vi "Illini Hyperloop GUI v4.0.vi"() -> ()   [LabVIEW 2015]
uses:
  CommunicationStatus.ctl
  <vilib>/robotics/Controls/Attitude Indicator/Attitude Indicator.xctl
  StageEnum.ctl
  ArxPaxGauge4.ctl
  MicrosecondsGauge1.ctl
panel:
  out "RPM Right Front":T1 scale=0.0..6000.0
  out "RPM Right Mid":T1 scale=0.0..6000.0
  out "LEV Micro":T2 scale=800.0..2000.0
  out "RPM Right Back":T1 scale=0.0..6000.0
  out "RPM Left Front":T1 scale=0.0..6000.0
  out "RPM Left Mid":T1 scale=0.0..6000.0
  out "LEV  Delay timer":dbl
  out "STA  Delay timer":dbl
  out "Battery Pack 2 V 2":dbl(slide) caption="Capacity %" scale=0.0..100.0
  out "Battery Pack 1 V 2":dbl(slide) caption="Capacity %" scale=0.0..100.0
  out "Battery Pack 2 V":dbl(slide) caption="Pack 2 (V)" scale=0.0..500.0
  out "Battery Pack 1 V":dbl(slide) caption="Pack 1 (V)" scale=0.0..500.0
  out "Levitation Chart":cluster{"element":dbl, "element":dbl}(graph)
  out "Braking Force Chart 1":dbl(slide) caption="Reservoir 1" scale=0.0..6000.0
  out "Levitation height front":dbl(slide) caption="Front" scale=0.0..20.0
  out "Levitation height back":dbl(slide) caption="Back" scale=0.0..20.0
  out "Current front right":dbl[unit] caption="Current"
  out "Voltage front right":dbl[unit] caption="Voltage"
  out "Current front left":dbl[unit] caption="Current"
  out "Voltage front left":dbl[unit] caption="Voltage"
  out "Current back right":dbl[unit] caption="Current"
  out "Voltage back right":dbl[unit] caption="Voltage"
  out "Current back left":dbl[unit] caption="Current"
  out "Voltage back left":dbl[unit] caption="Voltage"
  out "Attitude Indicator":cluster{"Roll":dbl, "Pitch":dbl}(xcontrol)
  out "Yaw":dbl(knob) scale=-15.0..15.0
  out "RPM Left Back":T1 scale=0.0..6000.0
  out "Cabin Pressure":dbl format="%#.3g"
  out "Ambient Pressure (psi)":dbl(graph)
  out "Pod State:":T3
  out "Communication Status:":T4
  out "Low Battery":dbl format="%#.2g"
  out "High Battery:":dbl format="%#.2g"
  out "Battery 3":dbl(slide) scale=0.0..100.0
  out "Battery 2":dbl(slide) scale=0.0..100.0
  out "Battery 1":dbl(slide) scale=0.0..100.0
  out "Z acc":dbl
  out "Y acc":dbl
  out "X acc":dbl
  out "Z vel":dbl
  out "Y vel":dbl
  out "X vel":dbl
  out "Z position":dbl
  out "Y pos":dbl
  out "X pos":dbl
  out "Velocity Chart":dbl(graph)
  in  "EMERGENCY BRAKE":bool
  in  "Functional Test Tab Control":T5(tab)
  out "Client Closed":string="The client VI closed the connection."
  out "Most Recent Data":string
  in  "Connect to":string="192.168.137.100"
  in  "timeout ms":i32=1000
  in  "port":u16=8888
  in  "ms per loop":u32
  in  "bytes per write":i32=1000
  out "Base File Name":string
  in  "Transition":bool
  in  "Transition to:":string(combo)="Safe Mode"
  out "bytes written":i32
  in  "Stop Program":bool
  out "Producer Error Messages":errorcluster
  out "Consumer Error Messages":errorcluster
  in  "LEV OFF":bool
  in  "STA Delay":dbl=100.0
  in  "LEV Delay":dbl=100.0
  in  "STA Start Stop":bool
  in  "LEV Start Stop":bool
  in  "STA jump Interval":dbl=5.0
  in  "STA Target":dbl=1000.0
  in  "LEV jump interval":dbl=5.0
  in  "LEV Target":dbl=1000.0
  in  "STA Init + Arm":bool
  in  "STA init":dbl
  in  "STA arm":dbl
  in  "LEV ON":bool
  in  "SET STA Manual":bool
  in  "Set LEV Manual":bool
  in  "LEV SLIDE":dbl(slide) scale=0.0..2000.0
  in  "STA Slide":dbl(slide) scale=0.0..2000.0
  in  "STA Margin":dbl=50.0
  in  "LEV Margin":dbl=50.0
  out "Functional Test C Data":string caption="Data:"
  in  "Functional Test 3":bool caption="Boolean"
  in  "Functional Test 4":bool caption="Boolean"
  out "Functional Test D Data":string caption="Data:"
  in  "Prepare for Launch":bool caption="Boolean"
  out "Acceleration Chart":dbl(graph)
  out "Checkmark":u16(ring)
  out "Position Chart":dbl(graph)
  out "Temperature other (C)":T6(graph)
  out "Temperature ESCs (C)":T7(graph)
  # "Illini Hyperloop"
  # "Brakes (PSI)"
  # "X Position (m)"
  # "Levitation (m)"
  # "Attitude"
  # "Levitation (mm)"
  # "X Acceleration (m/s/s)"
  # "X Velocity (m/s)"
  # "Levitation Battery Packs"
  # "Motor Control"
  # "Brake Control"
  # "Functional Test C: Communication Inside Tube"
  # "Functional Test D: Internal power and Levitation"
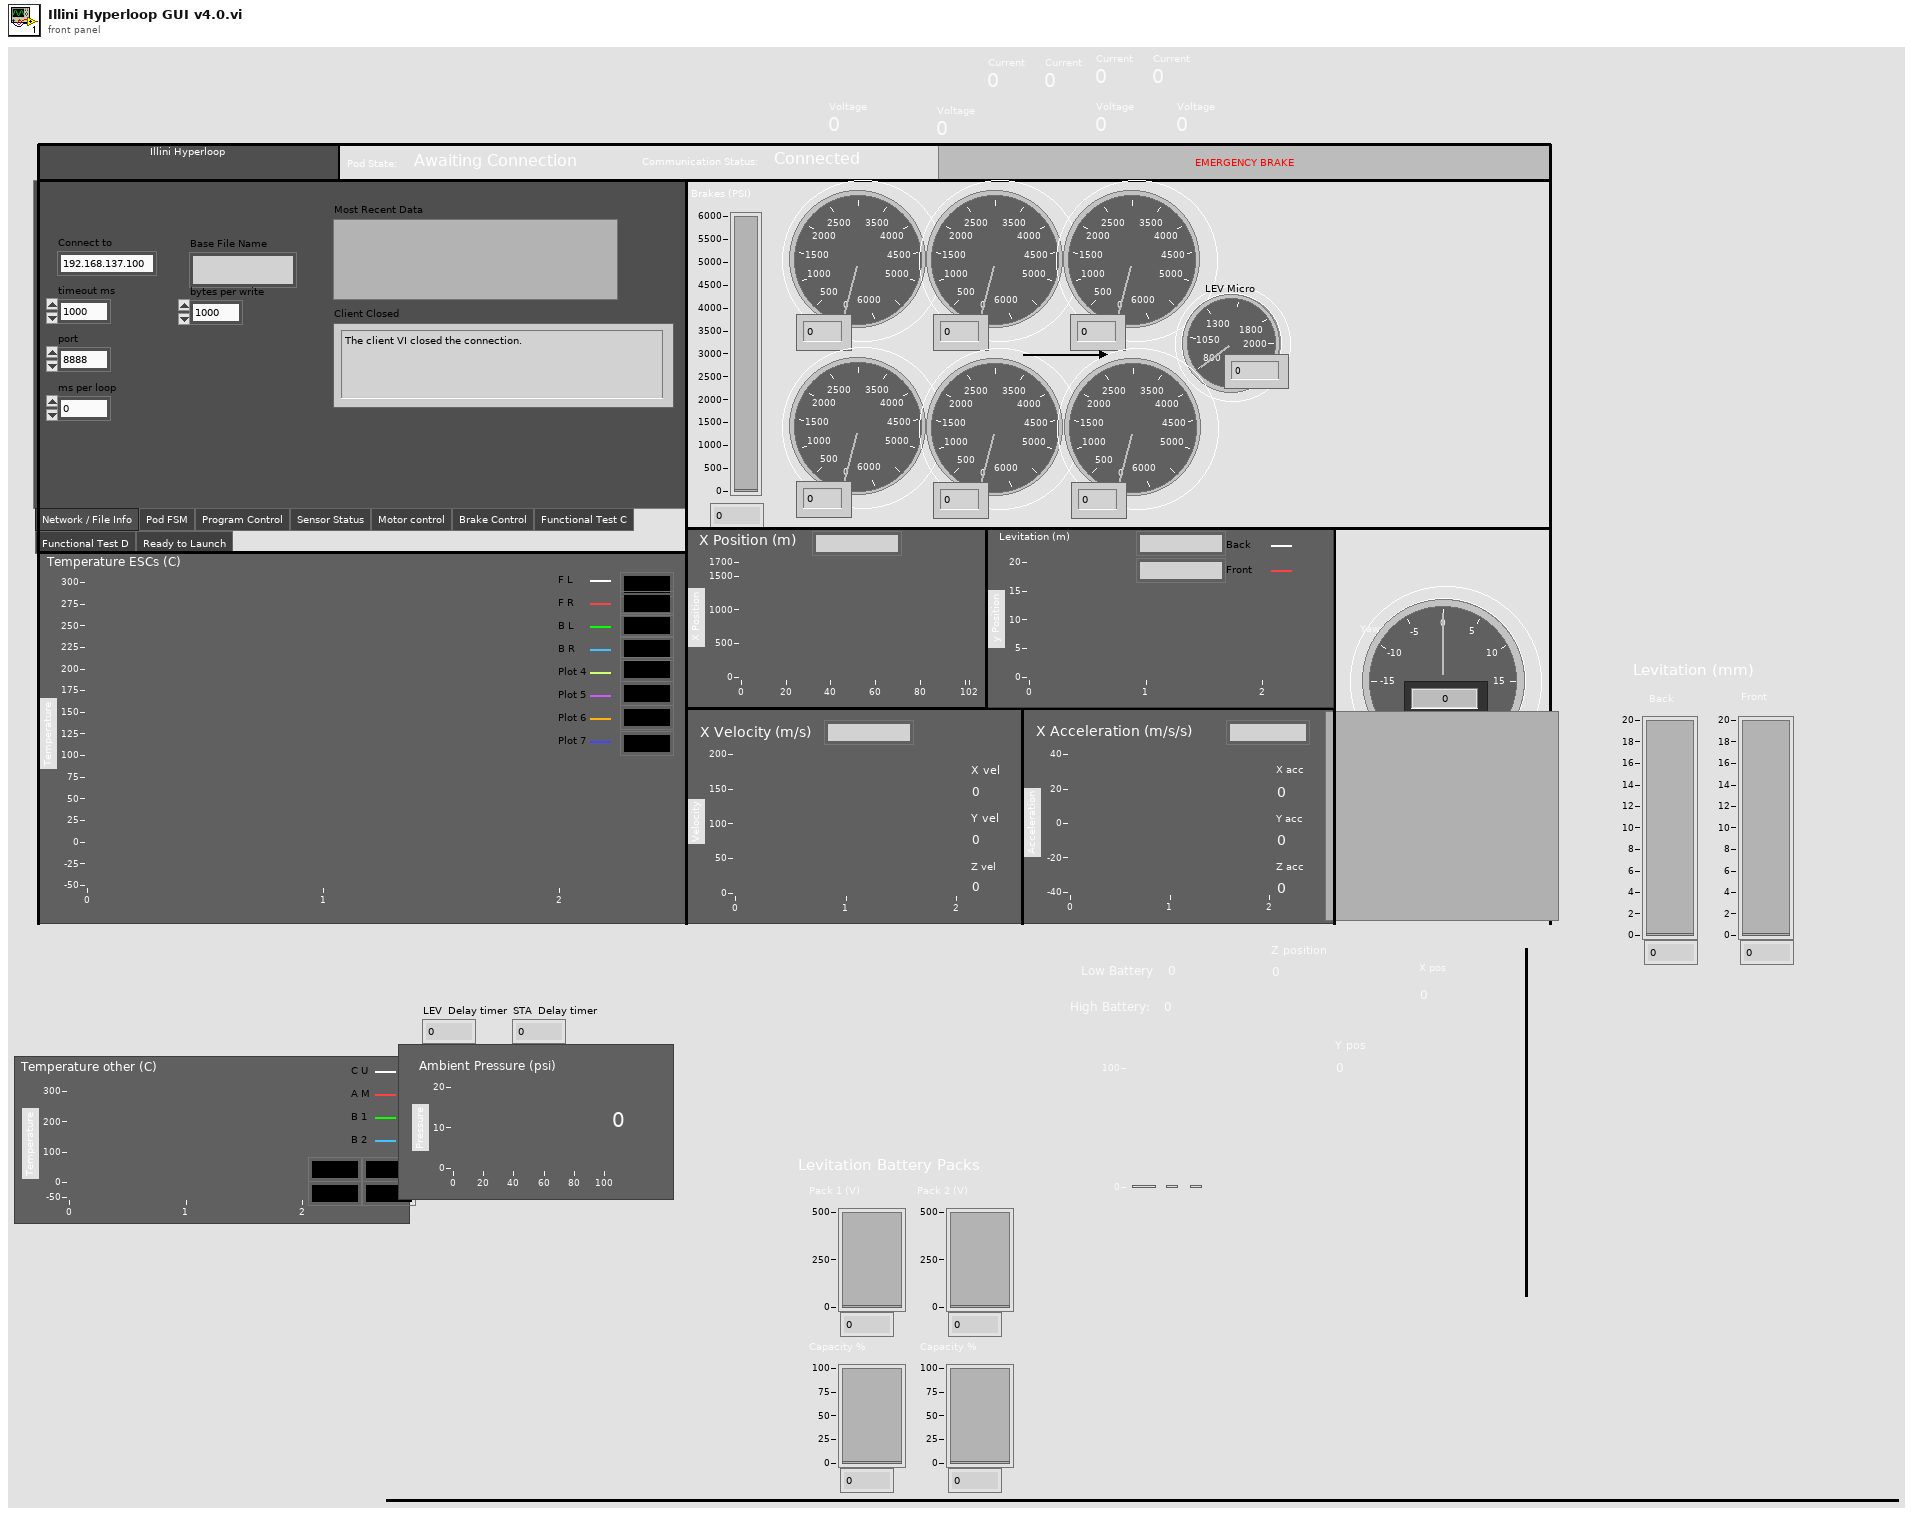
[diagram p1: front panel]
types:
  T1 = typedef "ArxPaxGauge4.ctl" = u32
  T2 = typedef "MicrosecondsGauge1.ctl" = dbl
  T3 = typedef "StageEnum.ctl" = enum16{"Awaiting Connection", "TEST Comms", "TEST Lev", "TEST Inside Comms", "TEST Internal Power", "Ready to Launch", "Acceleration", "Coast", "Brake"}
  T4 = typedef "CommunicationStatus.ctl" = enum16{"Connected", "Disconnected"}
  T5 = enum32{"Network / File Info", "Pod FSM", "Program Control", "Sensor Status", "Motor control", "Brake Control", "Functional Test C", "Functional Test D", "Ready to Launch"}
  T6 = cluster{"element":dbl, "element":dbl, "element":dbl, "element":dbl}
  T7 = cluster{"element":dbl, "element":dbl, "element":dbl, "element":dbl, "element":dbl, "element":dbl, "element":dbl, "element":dbl}
  T8 = cluster{"element":dbl, "element":dbl, "element":dbl, "element":dbl, "element":dbl, "element":dbl, "element":dbl, "element":dbl}[]
  T9 = cluster{"element":dbl, "element":dbl, "element":dbl, "element":dbl}[]
  T10 = enum16{"Standard", "Buffered", "CRLF", "Immediate"}
  T11 = cluster{i32, "data out":string, "data out":string}
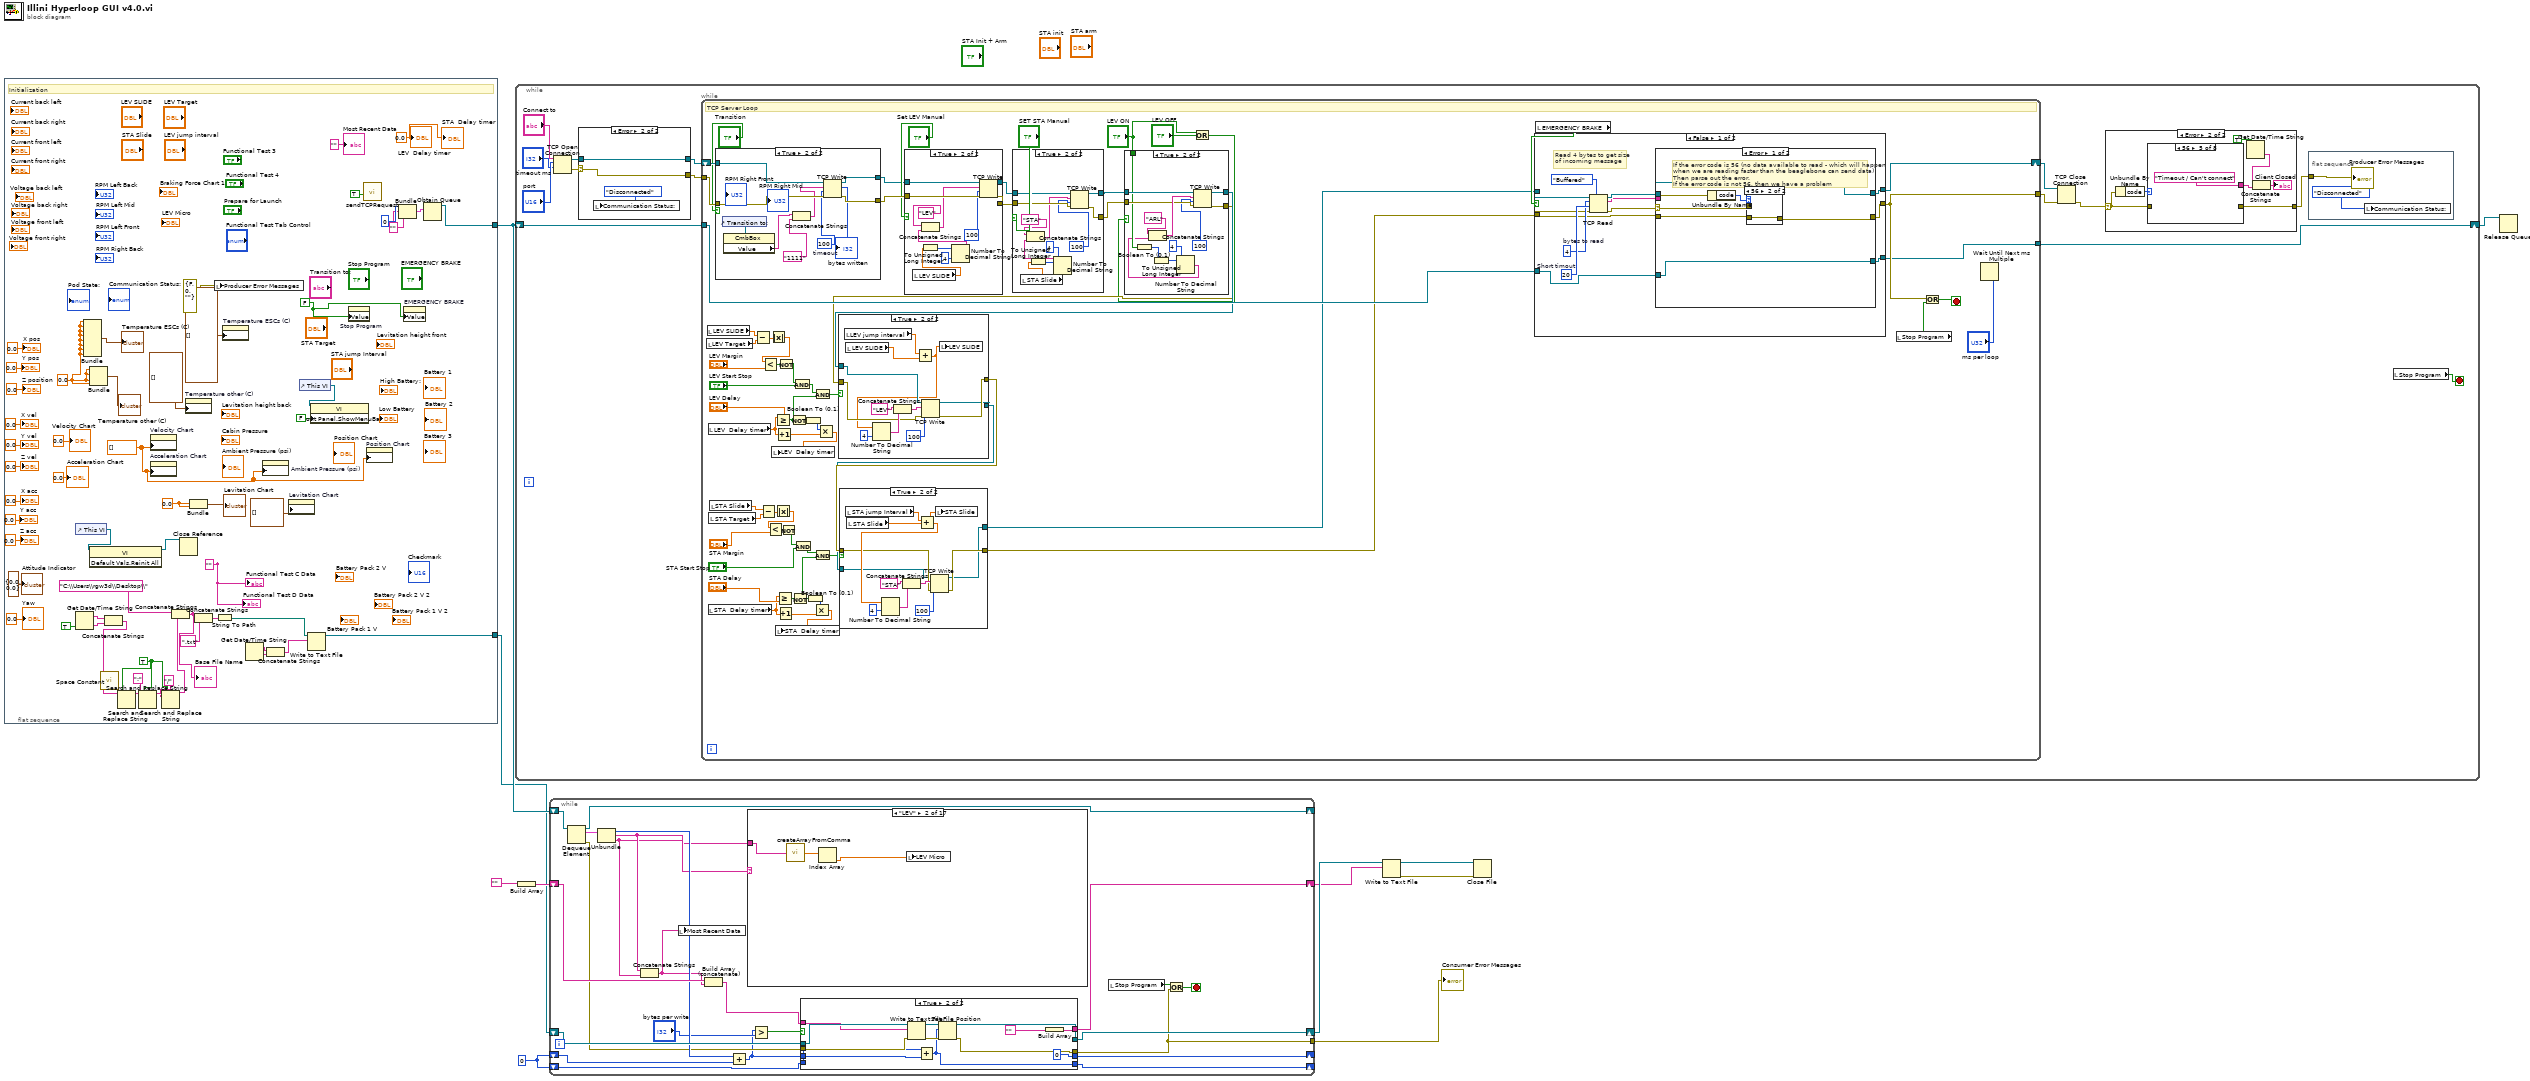
[diagram p0: block diagram]
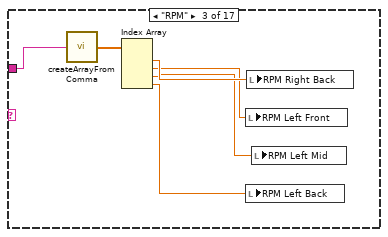
[diagram p4: hidden frame]
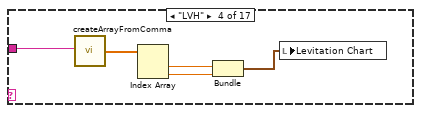
[diagram p5: hidden frame]
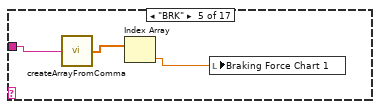
[diagram p6: hidden frame]
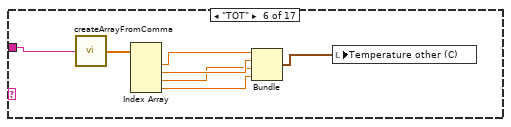
[diagram p7: hidden frame]
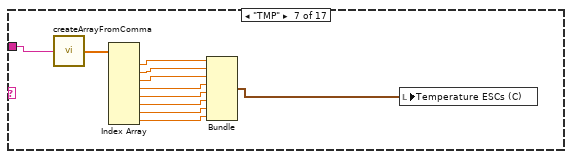
[diagram p8: hidden frame]
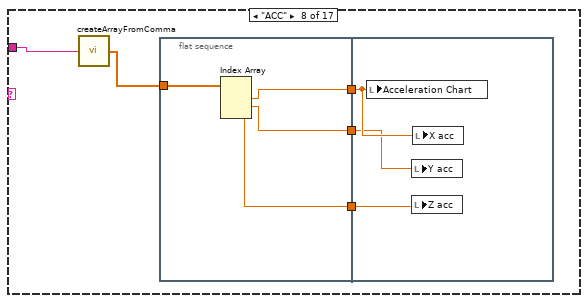
[diagram p9: hidden frame]
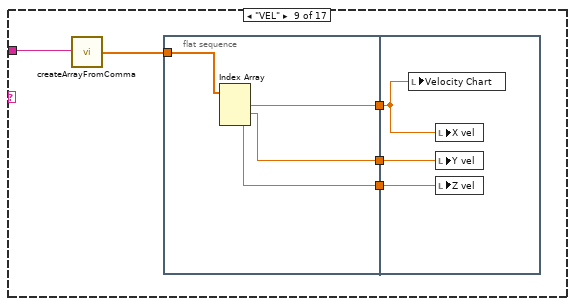
[diagram p10: hidden frame]
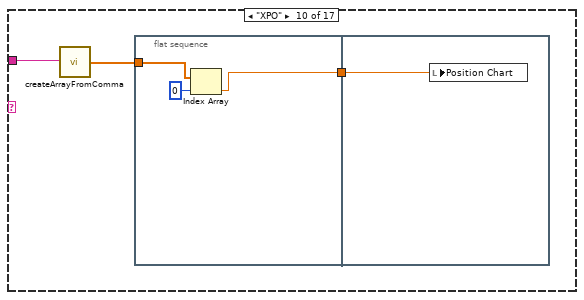
[diagram p11: hidden frame]
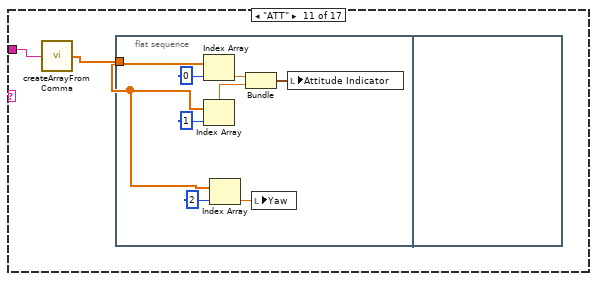
[diagram p12: hidden frame]
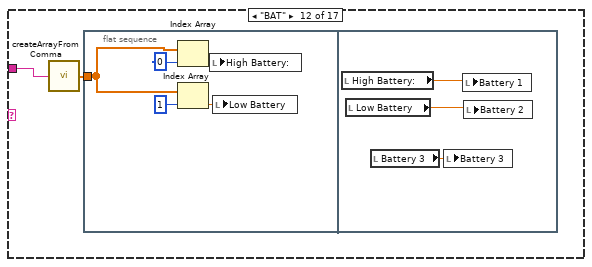
[diagram p13: hidden frame]
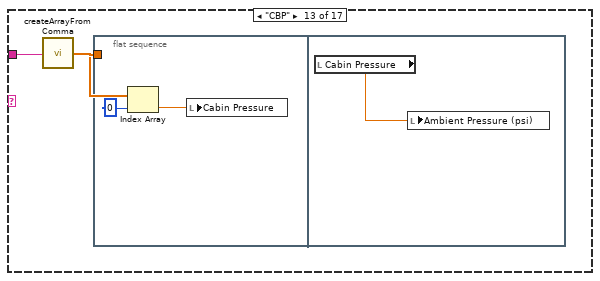
[diagram p14: hidden frame]
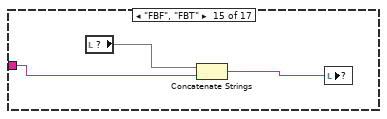
[diagram p16: hidden frame]
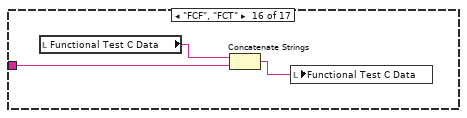
[diagram p17: hidden frame]
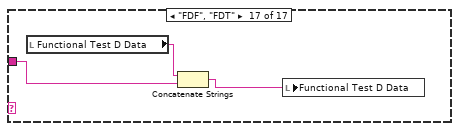
[diagram p18: hidden frame]
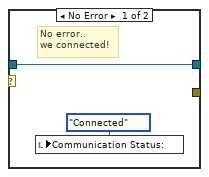
[diagram p19: hidden frame]
diagram:
  w1 = 0
  n1 = flat-sequence {
    tunnel: [w67] -> w11
    tunnel: [w40] -> w6
    frame #0 {
      w19 = 0.0 ("LEV  Delay timer")
      w23 = 0.0 ("element")
      w24 = TRUE ("want seconds? (F)")
      w37 = ""
      w44 = dbl[] [] ("History Data")
      w18 = 0.0 ("element")
      w52 = FALSE
      w20 = "" ("Functional Test 1 Data")
      # "Initialization"
      n2 = control-ref of="This VI"() -> (w46:refnum<vi>)
      n3 = Get Date/Time String(want seconds? (F)=TRUE) -> (date string=w35:string, time string=w34:string)  [unwired: 2 in]
      n4 = Bundle("element"=w18, "element"=w18, "element"=w18, "element"=w18, "element"=w18, "element"=w18, "element"=w18, "element"=w18) -> (→"Temperature ESCs (C)":T7)  [unwired: 1 in]
      n5 = Bundle("element"=w18, "element"=w18, "element"=w18, "element"=w18) -> (→"Temperature other (C)":T6)  [unwired: 1 in]
      n6 = invoke class="VI" method="Default Vals.Reinit All"(reference=w46) -> (reference out=w45:refnum<vi>)  [unwired: 2 in, 2 out]
      n7 = call <vilib>:"Space Constant.vi"() -> ("String"=w36:string)
      n8 = Concatenate Strings(w35, w34) -> (w33:string)
      n9 = Search and Replace String(replace all?=w24, input string=w33, search string=w36) -> (result string=w31:string)  [unwired: 5 in, 3 out]
      n10 = Search and Replace String(replace all?=w24, input string=w31, search string=":" ("Functional Test 1 Data")) -> (result string=w27:string)  [unwired: 5 in, 3 out]
      n11 = property on="Velocity Chart" class="WFChart (strict)"("History Data"=w44) -> ()  [unwired: 2 in, 2 out]
      n12 = property on="Acceleration Chart" class="WFChart (strict)"("History Data"=w44) -> ()  [unwired: 2 in, 2 out]
      n13 = Search and Replace String(replace all?=w24, input string=w27, search string="/" ("Functional Test 1 Data")) -> (result string=w26:string)  [unwired: 5 in, 3 out]
      n14 = Concatenate Strings("C:\\Users\\rgw3d\\Desktop\\" ("Functional Test 1 Data"), w26) -> (w13:string)
      "Base File Name" <- w13
      n15 = Close Reference(reference=w45) -> ()  [unwired: 1 in, 1 out]
      n16 = property on="Temperature other (C)" class="WFChart (strict)"("History Data"=T9 []) -> ()  [unwired: 2 in, 2 out]
      n17 = Bundle("element"=w23, "element"=w23) -> (→"Levitation Chart":cluster{"element":dbl, "element":dbl})  [unwired: 1 in]
      n18 = Concatenate Strings(w13, ".txt" ("Functional Test 1 Data")) -> (w14:string)
      n19 = local write "Producer Error Messages"(errorcluster {"status"=FALSE, "code"=0, "source"=""} ("error constant")) -> ()
      n20 = String To Path(string=w14) -> (path=w28:path)
      n21 = property on="Temperature ESCs (C)" class="WFChart (strict)"("History Data"=T8 []) -> ()  [unwired: 2 in, 2 out]
      n22 = Get Date/Time String() -> (date string=w43:string, time string=w42:string)  [unwired: 3 in]
      n23 = property on="Ambient Pressure (psi)" class="WFChart (strict)"("History Data"=w44) -> ()  [unwired: 2 in, 2 out]
      n24 = Concatenate Strings(w43, w42) -> (w41:string)
      n25 = property on="Levitation Chart" class="WFChart (strict)"("History Data"=cluster{"element":dbl, "element":dbl}[] []) -> ()  [unwired: 2 in, 2 out]
      n26 = control-ref of="This VI"() -> (w51:refnum<vi>)
      n27 = Write to Text File(file (use dialog)=w28, text=w41) -> (refnum out=w40:refnum<file>)  [unwired: 2 in, 2 out]
      n28 = property class="VI"(reference=w51, "Front Panel.ShowMenuBar"=FALSE ("Front Panel Window:Show Menu Bar")) -> ()  [unwired: 1 in, 2 out]
      n29 = property on="Stop Program" class="Bool (strict)"("Value"=w52) -> ()  [unwired: 2 in, 2 out]
      n30 = call "sendTCPRequest.vi"("Force Reset"=TRUE) -> ()  [unwired: 9 in, 2 out]
      n31 = property on="Position Chart" class="WFChart (strict)"("History Data"=w44) -> ()  [unwired: 2 in, 2 out]
      n32 = Bundle(0, w37, w37) -> (w39:cluster{i32, string, string})  [unwired: 1 in]
      n33 = property on="EMERGENCY BRAKE" class="Bool (strict)"("Value"=w52) -> ()  [unwired: 2 in, 2 out]
      n34 = Obtain Queue(element data type=w39) -> (queue out=w67:refnum<queue>)  [unwired: 4 in, 2 out]
      "X pos" <- 0.0 ("X position")
      "Y pos" <- 0.0 ("Y position")
      "Z position" <- 0.0 ("Z position")
      "X vel" <- 0.0 ("X velocity")
      "Y vel" <- 0.0 ("Y velocity")
      "Z vel" <- 0.0 ("Z velocity")
      "X acc" <- 0.0 ("X acceleration")
      "Y acc" <- 0.0 ("Y acceleration")
      "Z acc" <- 0.0 ("Z acceleration")
      "Velocity Chart" <- 0.0 ("Velocity (m/s)")
      "Attitude Indicator" <- cluster{"Roll":dbl, "Pitch":dbl} {"Roll"=0.0, "Pitch"=0.0} ("Attitude Indicator")
      "Acceleration Chart" <- 0.0 ("Acceleration Chart")
      "Yaw" <- 0.0 ("Yaw")
      "Functional Test C Data" <- w20
      "Functional Test D Data" <- w20
      "Most Recent Data" <- "" ("Data out")
      "LEV  Delay timer" <- w19
      "STA  Delay timer" <- w19
    }
  }
  n35 = while {
    shift-right: [w74] -> w10
    shift-left: w11 -> [w75]
    stop <- w71 stop-if-true
    n36 = TCP Open Connection(address="Connect to", remote port or service name="port", timeout ms (60000)="timeout ms") -> (connection ID=w76:refnum<k5>, error out=w77:errorcluster)  [unwired: 2 in]
    n37 = case shown="Error" w77 {
      selector: w77 -> [_ w87]
      tunnel: w76 -> [w85 w88]
      tunnel: [w85 w88] -> w69
      tunnel: [_ w87] -> w68
      frame No Error {
        # "No error.. \nwe connected!"
        n38 = local write "Communication Status:"(CommunicationStatus."Connected" ("Communication Status")) -> ()
      }
      frame Error {
        n39 = local write "Communication Status:"(CommunicationStatus."Disconnected" ("Communication Status")) -> ()
      }
    }
    n40 = while {
      tunnel: w68 -> [w160]
      tunnel: [w165] -> w73
      tunnel: w75 -> [w155]
      tunnel: [w164] -> w74
      shift-right: [w163] -> w70
      shift-left: w69 -> [w161]
      stop <- w154 stop-if-true
      # "TCP Server Loop"
      n41 = local read "LEV Target"() -> (w149:dbl)
      n42 = local read "LEV SLIDE"() -> (w150:dbl)
      n43 = local read "LEV  Delay timer"() -> (w133:dbl)
      n44 = local read "STA  Delay timer"() -> (w132:dbl)
      n45 = local read "STA Target"() -> (w143:dbl)
      n46 = local read "STA Slide"() -> (w144:dbl)
      n47 = case shown="True" "Transition" {
        tunnel: w161 -> [w237 w247]
        tunnel: w160 -> [w236 w245]
        tunnel: [w236 w244] -> w158
        tunnel: [w237 w246] -> w156
        frame False {
        }
        frame True {
          w243 = 100  # timeout
          n48 = control-ref of="Transition to:"() -> (w242:refnum<vi>)
          n49 = property class="CmbBox"(reference=w242) -> ("Value"=w240:string)  [unwired: 1 in, 2 out]
          n50 = Concatenate Strings(w240, "1111") -> (w238:string)
          n51 = TCP Write(connection ID=w247, data in=w238, error in (no error)=w245, 9:w243) -> (connection ID out=w246:refnum<k5>, bytes written=→"bytes written":i32, error out=w244:errorcluster)
        }
      }
      n52 = Subtract(x=w150, y=w149) -> (x-y=w148:dbl)
      n53 = Subtract(x=w144, y=w143) -> (x-y=w146:dbl)
      n54 = Absolute Value(x=w148) -> (abs(x)=w147:dbl)
      n55 = Less?(x=w147, y="LEV Margin") -> (x < y?=w124:bool)
      n56 = Greater Or Equal?(x=w133, y="LEV Delay") -> (x >= y?=w121:bool)
      n57 = Absolute Value(x=w146) -> (abs(x)=w145:dbl)
      n58 = Less?(x=w145, y="STA Margin") -> (x < y?=w115:bool)
      n59 = Increment(x=w133) -> (x+1=w130:dbl)
      n60 = Greater Or Equal?(x=w132, y="STA Delay") -> (x >= y?=w113:bool)
      n61 = Increment(x=w132) -> (x+1=w118:dbl)
      n62 = Not(x=w124) -> (.not. x?=w122:bool)
      n63 = Not(x=w115) -> (.not. x?=w116:bool)
      n64 = Not(x=w121) -> (.not. x?=w131:bool)
      n65 = Not(x=w113) -> (.not. x?=w126:bool)
      n66 = And(x=w122, y="LEV Start Stop") -> (x .and. y?=w120:bool)
      n67 = And(x=w116, y="STA Start Stop") -> (x .and. y?=w136:bool)
      n68 = Boolean To (0,1)(Boolean=w131) -> (0, 1=w128:i16)
      n69 = Boolean To (0,1)(Boolean=w126) -> (0, 1=w125:i16)
      n70 = Multiply(x=w125, y=w118) -> (x*y=w127:dbl)
      n71 = local write "STA  Delay timer"(w127) -> ()
      n72 = And(x=w120, y=w121) -> (x .and. y?=w134:bool)
      n73 = And(x=w136, y=w113) -> (x .and. y?=w135:bool)
      n74 = Multiply(x=w128, y=w130) -> (x*y=w129:dbl)
      n75 = local write "LEV  Delay timer"(w129) -> ()
      n76 = case shown="True" "Set LEV Manual" {
        tunnel: w158 -> [w223 w235]
        tunnel: [w223 w234] -> w152
        tunnel: w156 -> [w224 w233]
        tunnel: [w224 w232] -> w153
        frame False {
        }
        frame True {
          n77 = local read "LEV SLIDE"() -> (w226:dbl)
          n78 = To Unsigned Long Integer(number=w226) -> (unsigned 32bit integer=w225:u32)
          n79 = Number To Decimal String(number=w225, width (-)=i16 4) -> (decimal integer string=w229:string)
          n80 = Concatenate Strings("LEV", w229) -> (w228:string)
          n81 = TCP Write(connection ID=w233, data in=w228, error in (no error)=w235, 9:100 ("timeout ms (25000)")) -> (connection ID out=w232:refnum<k5>, error out=w234:errorcluster)  [unwired: 1 out]
        }
      }
      n82 = case shown="True" "SET STA Manual" {
        tunnel: w153 -> [w211 w222]
        tunnel: [w211 w221] -> w112
        tunnel: w152 -> [w210 w220]
        tunnel: [w210 w219] -> w111
        frame False {
        }
        frame True {
          n83 = local read "STA Slide"() -> (w212:dbl)
          n84 = To Unsigned Long Integer(number=w212) -> (unsigned 32bit integer=w213:u32)
          n85 = Number To Decimal String(number=w213, width (-)=i16 4) -> (decimal integer string=w216:string)
          n86 = Concatenate Strings("STA", w216) -> (w215:string)
          n87 = TCP Write(connection ID=w222, data in=w215, error in (no error)=w220, 9:100 ("timeout ms (25000)")) -> (connection ID out=w221:refnum<k5>, error out=w219:errorcluster)  [unwired: 1 out]
        }
      }
      n88 = Or(x="LEV ON", y="LEV OFF") -> (x .or. y?=w107:bool)
      n89 = case shown="True" w107 {
        tunnel: w112 -> [w168 w178]
        tunnel: w111 -> [w169 w177]
        tunnel: [w169 w176] -> w109
        tunnel: [w168 w175] -> w110
        tunnel: "LEV ON" -> [_ w172]
        frame False {
        }
        frame True {
          n90 = Boolean To (0,1)(Boolean=w172) -> (0, 1=w173:i16)
          n91 = To Unsigned Long Integer(number=w173) -> (unsigned 32bit integer=w179:u32)
          n92 = Number To Decimal String(number=w179, width (-)=i16 4) -> (decimal integer string=w170:string)
          n93 = Concatenate Strings("ARL", w170) -> (w181:string)
          n94 = TCP Write(connection ID=w178, data in=w181, error in (no error)=w177, 9:100 ("timeout ms (25000)")) -> (connection ID out=w175:refnum<k5>, error out=w176:errorcluster)  [unwired: 1 out]
        }
      }
      n95 = case shown="True" w134 {
        tunnel: w110 -> [w197 w203]
        tunnel: [w197 w199] -> w140
        tunnel: w109 -> [w196 w202]
        tunnel: [w196 w201] -> w142
        frame False {
        }
        frame True {
          n96 = local read "LEV jump interval"() -> (w209:dbl)
          n97 = local read "LEV SLIDE"() -> (w208:dbl)
          n98 = Add(x=w209, y=w208) -> (x+y=w200:dbl)
          n99 = Number To Decimal String(number=w200, width (-)=i16 4) -> (decimal integer string=w205:string)
          n100 = Concatenate Strings("LEV", w205) -> (w207:string)
          n101 = TCP Write(connection ID=w203, data in=w207, error in (no error)=w202, 9:100 ("timeout ms (25000)")) -> (connection ID out=w199:refnum<k5>, error out=w201:errorcluster)  [unwired: 1 out]
          n102 = local write "LEV SLIDE"(w200) -> ()
        }
      }
      n103 = case shown="True" w135 {
        tunnel: w142 -> [w183 w187]
        tunnel: [w183 w186] -> w141
        tunnel: w140 -> [w182 w185]
        tunnel: [w182 w184] -> w139
        frame False {
        }
        frame True {
          n104 = local read "STA jump Interval"() -> (w195:dbl)
          n105 = local read "STA Slide"() -> (w194:dbl)
          n106 = Add(x=w195, y=w194) -> (x+y=w188:dbl)
          n107 = Number To Decimal String(number=w188, width (-)=i16 4) -> (decimal integer string=w191:string)
          n108 = Concatenate Strings("STA", w191) -> (w193:string)
          n109 = TCP Write(connection ID=w185, data in=w193, error in (no error)=w187, 9:100 ("timeout ms (25000)")) -> (connection ID out=w184:refnum<k5>, error out=w186:errorcluster)  [unwired: 1 out]
          n110 = local write "STA Slide"(w188) -> ()
        }
      }
      n111 = local read "EMERGENCY BRAKE"() -> (w167:bool)
      n112 = case shown="False" w167 {
        tunnel: w141 -> [w256 w281]
        tunnel: w139 -> [w257 w280]
        tunnel: [w253 w279] -> w163
        tunnel: [w249 w278] -> w165
        tunnel: w155 -> [w251 w277]
        tunnel: [w250 w277] -> w164
        frame False {
          w258 = 4  # bytes to read
          w259 = 20  # Short timout
          # "Read 4 bytes to get size\nof incoming message"
          n113 = TCP Read(connection ID=w257, bytes to read=w258, error in (no error)=w256, 7:T10."Buffered" ("mode (standard)"), 9:w259) -> (connection ID out=w254:refnum<k5>, data out=w252:string, error out=w255:errorcluster)
          n114 = case shown="Error" w255 {
            selector: w255 -> [w263 _]
            tunnel: w256 -> [w264 w274]
            tunnel: [w262 w269] -> w249
            tunnel: w254 -> [w261 w275]
            tunnel: [w261 w273] -> w253
            tunnel: w252 -> [_ w276]
            tunnel: w251 -> [w260 w271]
            tunnel: [w260 w268] -> w250
            frame Error {
              # "If the error code is 56 (no data available to read - which will happen when we are reading faster than the beaglebone can send data) Then parse out the error. \nIf the error code is not 56, then we have a problem"
              n115 = Unbundle By Name(w263) -> ("code"=w265:i32)
              n116 = case shown="56" w265 {
                tunnel: w263 -> [w266 _]
                tunnel: [w266 w267] -> w262
                tunnel: w264 -> [_ w267]
                frame Default {
                }
                frame 56 {
                }
              }
            }
            frame No Error {
              n117 = call "readTCPDataIn v1.vi"("TCP Network Connection in"=w275, "Size of data"=w276, "error in (no error)"=w274) -> ("TCP Network Connection out"=w273:refnum<k5>, "Size+Operation+Data"=w272:T11, "error out"=w270:errorcluster)  [unwired: 8 in, 2 out]
              n118 = Enqueue Element(queue=w271, element=w272, error in (no error)=w270) -> (queue out=w268:refnum<queue>, error out=w269:errorcluster)  [unwired: 1 in, 1 out]
            }
          }
        }
        frame True {
          n119 = TCP Write(connection ID=w280, data in="OFF0000", error in (no error)=w281) -> (connection ID out=w279:refnum<k5>, error out=w278:errorcluster)  [unwired: 1 in, 1 out]
        }
      }
      n120 = local read "Stop Program"() -> (w166:bool)
      n121 = Or(x=w165, y=w166) -> (x .or. y?=w154:bool)
      n122 = Wait Until Next ms Multiple(millisecond multiple="ms per loop") -> ()  [unwired: 1 out]
    }
    n123 = TCP Close Connection(connection ID=w70, error in (no error)=w73) -> (error out=w81:errorcluster)  [unwired: 2 out]
    n124 = case shown="Error" w81 {
      selector: w81 -> [w89 w95]
      tunnel: [w89 w94] -> w80
      frame No Error {
      }
      frame Error {
        n125 = Unbundle By Name(w95) -> ("code"=w96:i32)
        n126 = case shown="56" w96 {
          tunnel: w95 -> [_ _ w100 _ _ _ _ _]
          tunnel: [_ _ w100 _ _ _ _ _] -> w94
          tunnel: ["The network is down, \nunreachable, or has been reset." "The specified network \naddress is currently in use." "Error" "The system caused the network \nconnection to be aborted." "Timeout / Can't connect" "Error 63. LabVIEW: The network connection \nwas refused by the server." "\tThe network connection\n is not yet established." "The network connection\n was closed by the peer."] -> w91
          frame 59 {
          }
          frame 60 {
          }
          frame Default {
          }
          frame 62 {
          }
          frame 56 {
          }
          frame 63 {
          }
          frame 64 {
          }
          frame 66 {
          }
        }
        n127 = Get Date/Time String(want seconds? (F)=TRUE) -> (time string=w92:string)  [unwired: 2 in, 1 out]
        n128 = Concatenate Strings(w92, w91) -> (→"Client Closed":string)
      }
    }
    n129 = flat-sequence {
      tunnel: w80 -> [w83]
      frame #0 {
        n130 = local write "Communication Status:"(CommunicationStatus."Disconnected" ("Communication Status")) -> ()
        "Producer Error Messages" <- w83
      }
    }
    n131 = local read "Stop Program"() -> (w71:bool)
  }
  n132 = Build Array("") -> (w7:string[])
  n133 = while {
    shift-right: [w305] -> _
    shift-left: w11 -> [w304]
    tunnel: [w293] -> w9
    shift-right: [w285] -> w2
    shift-left: w7 -> [w301]
    shift-right: [w299] -> w5
    shift-left: w6 -> [w300]
    shift-right: [w292] -> _
    shift-left: w1 -> [w296]
    shift-right: [w283] -> _
    shift-left: w1 -> [w284]
    stop <- w302 stop-if-true
    n134 = Dequeue Element(queue=w304) -> (queue out=w305:refnum<queue>, element=w298:cluster{i32, string, string}, error out=w295:errorcluster)  [unwired: 2 in, 1 out]
    n135 = Unbundle(w298) -> (w297:i32, w291:string, w290:string)
    n136 = Concatenate Strings(w291, w290) -> (w288:string)
    n137 = local write "Most Recent Data"(w288) -> ()
    n138 = Build Array (concatenate)(w301, w288) -> (w287:string[])
    n139 = Add(x=w297, y=w296) -> (x+y=w286:i32)
    n140 = case shown="\"LEV\"" w291 {
      tunnel: w290 -> [_ w325 w331 w337 w340 w341 w358 w363 w375 w385 w391 w400 w410 _ w416 w419 w422]
      frame Default {
      }
      frame "LEV" {
        n141 = call "createArrayFromComma.vi"("String"=w325) -> ("Array"=w326:dbl[])
        n142 = Index Array(array=w326) -> (element=w324:dbl)  [unwired: 1 in]
        n143 = local write "LEV Micro"(w324) -> ()
      }
      frame "RPM" {
        n144 = call "createArrayFromComma.vi"("String"=w331) -> ("Array"=w332:dbl[])
        n145 = Index Array(array=w332) -> (element #1=w330:dbl, element #2=w329:dbl, element #3=w328:dbl, element #4=w327:dbl)  [unwired: 4 in]
        n146 = local write "RPM Left Front"(w329) -> ()
        n147 = local write "RPM Left Back"(w327) -> ()
        n148 = local write "RPM Right Back"(w330) -> ()
        n149 = local write "RPM Left Mid"(w328) -> ()
      }
      frame "LVH" {
        n150 = call "createArrayFromComma.vi"("String"=w337) -> ("Array"=w336:dbl[])
        n151 = Index Array(array=w336) -> (element #1=w335:dbl, element #2=w334:dbl)  [unwired: 2 in]
        n152 = Bundle(w335, w334) -> (w333:cluster{dbl, dbl})  [unwired: 1 in]
        n153 = local write "Levitation Chart"(w333) -> ()
      }
      frame "BRK" {
        n154 = call "createArrayFromComma.vi"("String"=w340) -> ("Array"=w339:dbl[])
        n155 = Index Array(array=w339) -> (element=w338:dbl)  [unwired: 1 in]
        n156 = local write "Braking Force Chart 1"(w338) -> ()
      }
      frame "TOT" {
        n157 = call "createArrayFromComma.vi"("String"=w341) -> ("Array"=w347:dbl[])
        n158 = Index Array(array=w347) -> (element #1=w346:dbl, element #2=w345:dbl, element #3=w344:dbl, element #4=w343:dbl)  [unwired: 4 in]
        n159 = Bundle(w346, w345, w344, w343) -> (w342:cluster{dbl, dbl, dbl, dbl})  [unwired: 1 in]
        n160 = local write "Temperature other (C)"(w342) -> ()
      }
      frame "TMP" {
        n161 = call "createArrayFromComma.vi"("String"=w358) -> ("Array"=w357:dbl[])
        n162 = Index Array(array=w357) -> (element #1=w356:dbl, element #2=w355:dbl, element #3=w353:dbl, element #4=w352:dbl, element #5=w351:dbl, element #6=w350:dbl, element #7=w349:dbl, element #8=w348:dbl)  [unwired: 8 in]
        n163 = Bundle(w356, w355, w353, w352, w351, w350, w349, w348) -> (w354:cluster{dbl, dbl, dbl, dbl, dbl, dbl, dbl, dbl})  [unwired: 1 in]
        n164 = local write "Temperature ESCs (C)"(w354) -> ()
      }
      frame "ACC" {
        n165 = call "createArrayFromComma.vi"("String"=w363) -> ("Array"=w362:dbl[])
        n166 = flat-sequence {
          tunnel: w362 -> [w367]
          tunnel: [w366] -> w361
          tunnel: [w365] -> w360
          tunnel: [w364] -> w359
          tunnel: w361 -> [w370]
          tunnel: w360 -> [w369]
          tunnel: w359 -> [w368]
          frame #0 {
            n167 = Index Array(array=w367) -> (element #1=w366:dbl, element #2=w365:dbl, element #3=w364:dbl)  [unwired: 3 in]
          }
          frame #1 {
            n168 = local write "Acceleration Chart"(w370) -> ()
            n169 = local write "Y acc"(w369) -> ()
            n170 = local write "Z acc"(w368) -> ()
            n171 = local write "X acc"(w370) -> ()
          }
        }
      }
      frame "VEL" {
        n172 = call "createArrayFromComma.vi"("String"=w375) -> ("Array"=w374:dbl[])
        n173 = flat-sequence {
          tunnel: w374 -> [w379]
          tunnel: [w378] -> w373
          tunnel: [w377] -> w372
          tunnel: [w376] -> w371
          tunnel: w373 -> [w382]
          tunnel: w372 -> [w381]
          tunnel: w371 -> [w380]
          frame #0 {
            n174 = Index Array(array=w379) -> (element #1=w378:dbl, element #2=w377:dbl, element #3=w376:dbl)  [unwired: 3 in]
          }
          frame #1 {
            n175 = local write "Velocity Chart"(w382) -> ()
            n176 = local write "X vel"(w382) -> ()
            n177 = local write "Y vel"(w381) -> ()
            n178 = local write "Z vel"(w380) -> ()
          }
        }
      }
      frame "XPO" {
        n179 = call "createArrayFromComma.vi"("String"=w385) -> ("Array"=w384:dbl[])
        n180 = flat-sequence {
          tunnel: w384 -> [w387]
          tunnel: [w386] -> w383
          tunnel: w383 -> [w389]
          frame #0 {
            n181 = Index Array(array=w387, index=0) -> (element=w386:dbl)
          }
          frame #1 {
            n182 = local write "Position Chart"(w389) -> ()
          }
        }
      }
      frame "ATT" {
        n183 = call "createArrayFromComma.vi"("String"=w391) -> ("Array"=w390:dbl[])
        n184 = flat-sequence {
          tunnel: w390 -> [w392]
          frame #0 {
            n185 = Index Array(array=w392, index=0) -> (element=w396:dbl)
            n186 = Index Array(array=w392, index=1) -> (element=w395:dbl)
            n187 = Index Array(array=w392, index=2) -> (element=w393:dbl)
            n188 = Bundle(w396, w395) -> (w394:cluster{dbl, dbl})  [unwired: 1 in]
            n189 = local write "Yaw"(w393) -> ()
            n190 = local write "Attitude Indicator"(w394) -> ()
          }
          frame #1 {
          }
        }
      }
      frame "BAT" {
        n191 = call "createArrayFromComma.vi"("String"=w400) -> ("Array"=w401:dbl[])
        n192 = flat-sequence {
          tunnel: w401 -> [w402]
          frame #0 {
            n193 = Index Array(array=w402, index=0) -> (element=w404:dbl)
            n194 = Index Array(array=w402, index=1) -> (element=w403:dbl)
            n195 = local write "High Battery:"(w404) -> ()
            n196 = local write "Low Battery"(w403) -> ()
          }
          frame #1 {
            n197 = local read "High Battery:"() -> (w408:dbl)
            n198 = local read "Low Battery"() -> (w409:dbl)
            n199 = local read "Battery 3"() -> (w407:dbl)
            n200 = local write "Battery 3"(w407) -> ()
            n201 = local write "Battery 1"(w408) -> ()
            n202 = local write "Battery 2"(w409) -> ()
          }
        }
      }
      frame "CBP" {
        n203 = call "createArrayFromComma.vi"("String"=w410) -> ("Array"=w411:dbl[])
        n204 = flat-sequence {
          tunnel: w411 -> [w413]
          frame #0 {
            n205 = Index Array(array=w413, index=0) -> (element=w412:dbl)
            n206 = local write "Cabin Pressure"(w412) -> ()
          }
          frame #1 {
            n207 = local read "Cabin Pressure"() -> (w415:dbl)
            n208 = local write "Ambient Pressure (psi)"(w415) -> ()
          }
        }
      }
      frame "FAF", "FAT" {
      }
      frame "FBF", "FBT" {
        n209 = local read item#-1() -> (w418)
        n210 = Concatenate Strings(w418, w416) -> (w417:string)
        n211 = local write item#-1(w417) -> ()
      }
      frame "FCF", "FCT" {
        n212 = local read "Functional Test C Data"() -> (w421:string)
        n213 = Concatenate Strings(w421, w419) -> (w420:string)
        n214 = local write "Functional Test C Data"(w420) -> ()
      }
      frame "FDF", "FDT" {
        n215 = local read "Functional Test D Data"() -> (w423:string)
        n216 = Concatenate Strings(w423, w422) -> (w424:string)
        n217 = local write "Functional Test D Data"(w424) -> ()
      }
    }
    n218 = Greater?(x=w286, y="bytes per write") -> (0:w294:bool)
    n219 = case shown="True" w294 {
      tunnel: w287 -> [w307 w314]
      tunnel: w300 -> [w310 w323]
      tunnel: [w310 w317] -> w299
      tunnel: w286 -> [w309 w312]
      tunnel: [w308 w320] -> w293
      tunnel: w295 -> [w308 w319]
      tunnel: [w309 0] -> w292
      tunnel: [w307 w315] -> w285
      tunnel: w284 -> [w306 w313]
      tunnel: [w306 w311] -> w283
      frame False {
      }
      frame True {
        n220 = Write to Text File(file (use dialog)=w323, text=w314, error in=w319) -> (refnum out=w322:refnum<file>, error out=w321:errorcluster)  [unwired: 1 in, 1 out]
        n221 = Add(x=w313, y=w312) -> (x+y=w311:i32)
        n222 = Set File Position(offset (in bytes) (0)=w311, refnum=w322, error in=w321) -> (refnum out=w317:refnum<file>, error out=w320:errorcluster)  [unwired: 1 in]
        n223 = Build Array("") -> (w315:string[])
      }
    }
    n224 = local read "Stop Program"() -> (w303:bool)
    n225 = Or(x=w303, y=w293) -> (x .or. y?=w302:bool)
  }
  "Consumer Error Messages" <- w9
  n226 = Write to Text File(file (use dialog)=w5, text=w2) -> (refnum out=w3:refnum<file>, error out=w4:errorcluster)  [unwired: 2 in, 1 out]
  n227 = Close File(refnum=w3, error in=w4) -> ()  [unwired: 2 out]
  n228 = Release Queue(queue=w10) -> ()  [unwired: 2 in, 3 out]
